vi "configure.vi"(8 "error in (no error)":errorcluster, 11 "ILCSim1TC in":refnum<class "ILCSim1TC.lvclass">) -> (0 "error out":errorcluster, 3 "ILCSim1TC out":refnum<class "ILCSim1TC.lvclass">)   [LabVIEW 2015, in "ILCSim1TC.lvclass"]
uses:
  ILCSim1TC.lvclass
  <userlib>/Common/ILC/Configuration/ILCADC.ctl
  <userlib>/Common/Simulators/ILCSim1/ILCSim1.lvclass/ILCSim1.ctl
  ConfigurationThisComponent/ConfigurationThisComponent.lvclass
  <userlib>/Common/ILC/Configuration/ILCConfiguration.lvlib
  <userlib>/Common/Simulators/ILCSim1/ILCSim1.lvclass
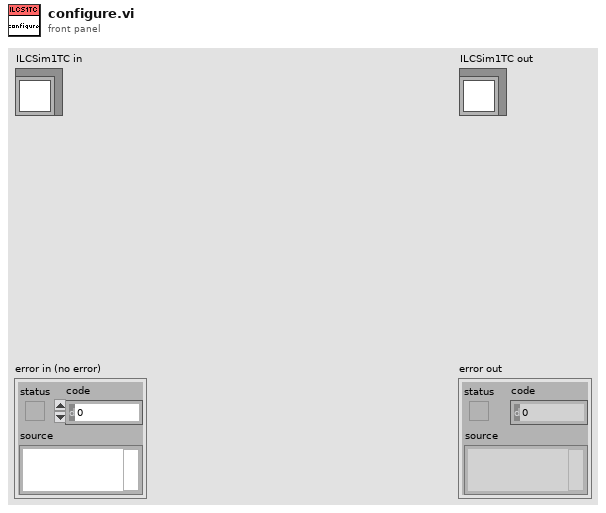
[diagram p1: front panel]
types:
  T1 = typedef "ILCCommon.lvlib/ILCConfiguration.lvlib/ILCADC.ctl" = cluster{"Reference Voltage Vref":dbl[unit], "Nominal Input Range in Counts":u32, "Preamplifier Gain":u8, "Conversion Settling Cycles":u16}
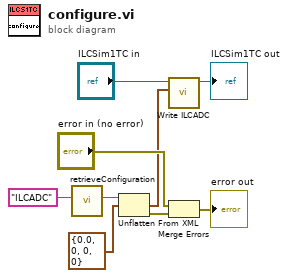
[diagram p0: block diagram]
diagram:
  n1 = call "retrieveConfiguration.vi"("configName"="ILCADC") -> ("xmlConfig"=w8:string)  [unwired: 8 in, 2 out]
  n2 = Unflatten From XML(xml string=w8, type=T1 {"Reference Voltage Vref"=0.0, "Nominal Input Range in Counts"=0, "Preamplifier Gain"=0, "Conversion Settling Cycles"=0} ("ILCADC")) -> (value=w2:T1, error out=w7:errorcluster)  [unwired: 1 in]
  n3 = call <userlib>:"Write ILCADC.vi"("ILC ADC"=w2, "ILCSim1 in"="ILCSim1TC in") -> ("ILCSim1 out"=→"ILCSim1TC out":refnum<class "ILCSim1TC.lvclass">)  [unwired: 9 in]
  n4 = Merge Errors("error in (no error)", w7) -> (→"error out":errorcluster)
